vi "LM34CAZ.vi"(11 "voltage":dbl=0.79 format="%#_13g") -> (0 "CJC (K)":dbl, 1 "CJC (C)":dbl, 2 "CJC (F)":dbl, 3 "CJC (V)":dbl)   [LabVIEW 2019]
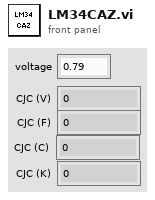
[diagram p1: front panel]
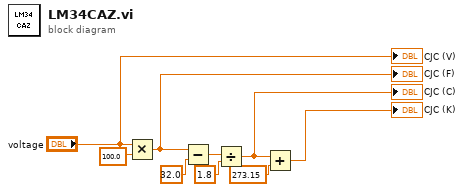
[diagram p0: block diagram]
diagram:
  n1 = Multiply(x="voltage", y=100.0) -> (x*y=w5:dbl)
  "CJC (F)" <- w5
  n2 = Subtract(x=w5, y=32.0) -> (x-y=w9:dbl)
  n3 = Divide(x=w9, y=1.8) -> (x/y=w2:dbl)
  "CJC (C)" <- w2
  n4 = Add(x=w2, y=273.15) -> (x+y=→"CJC (K)":dbl)
  "CJC (V)" <- "voltage"
